vi "process speedline data.vi"(8 "Cluster in":T1={"rigChannels"=[], "rigUnits"=[], "logging"=FALSE, "chartRef"=refnum, "dataTableRef"=refnum, "channelCount"=0, "trendIndex"=0, "channels"={"massflow"=0, "PR"=0, "recircTemp"=0}, "History"={"speedlines"=[], "liveTail"={"mDot"=[], "pRatio"=[]}, "current"={"mDot"=0.0, "pRatio"=0.0}, "insertPoint"=0, "tempHistory"=[]}, "filter"=FALSE, "filterLength"=0, "tableUpdate"=0, "limitValues"=[[0.0, 45000.0], [0.0, 100.0], [0.0, 100.0], [10.0, 100.0], [0.0, 100.0], [10.0, 35.0], [0.0, 100.0], [0.0, 100.0], [99000.0, 300000.0], [-5000.0, 5000.0], [99000.0, 300000.0], [-0.01, 0.3], [-0.01, 4.5], [-0.1, 100.0], [1.0, 8.0], [1.0, 5.0], [0.0, 100.0], [0.0, 100.0], [0.0, 100.0], [-100.0, 45000.0], [-0.1, 1.0], [0.8, 2.0], [90000.0, 110000.0], [15.0, 35.0], [0.0, 0.0], [0.0, 0.0], [0.0, 0.0], [0.0, 0.0]]}, 11 "data":variant) -> (0 "Cluster out":T1={"rigChannels"=[], "rigUnits"=[], "logging"=FALSE, "chartRef"=refnum, "dataTableRef"=refnum, "channelCount"=0, "trendIndex"=0, "channels"={"massflow"=0, "PR"=0, "recircTemp"=0}, "History"={"speedlines"=[], "liveTail"={"mDot"=[], "pRatio"=[]}, "current"={"mDot"=0.0, "pRatio"=0.0}, "insertPoint"=0, "tempHistory"=[]}, "filter"=FALSE, "filterLength"=0, "tableUpdate"=0, "limitValues"=[[0.0, 45000.0], [0.0, 100.0], [0.0, 100.0], [10.0, 100.0], [0.0, 100.0], [10.0, 35.0], [0.0, 100.0], [0.0, 100.0], [99000.0, 300000.0], [-5000.0, 5000.0], [99000.0, 300000.0], [-0.01, 0.3], [-0.01, 4.5], [-0.1, 100.0], [1.0, 8.0], [1.0, 5.0], [0.0, 100.0], [0.0, 100.0], [0.0, 100.0], [-100.0, 45000.0], [-0.1, 1.0], [0.8, 2.0], [90000.0, 110000.0], [15.0, 35.0], [0.0, 0.0], [0.0, 0.0], [0.0, 0.0], [0.0, 0.0]]}, 1 "updateTable":bool, 2 "dataTable":string[][](table), 3 "plotData":cluster{"pRatio":dbl[], "mDot":dbl[]}[](array[cluster]), 4 "Recirculation Delta":dbl, 5 "temp history":dbl[][](array[numeric]))   [LabVIEW 2018]
uses:
  custom sub vis/speedlineData.ctl
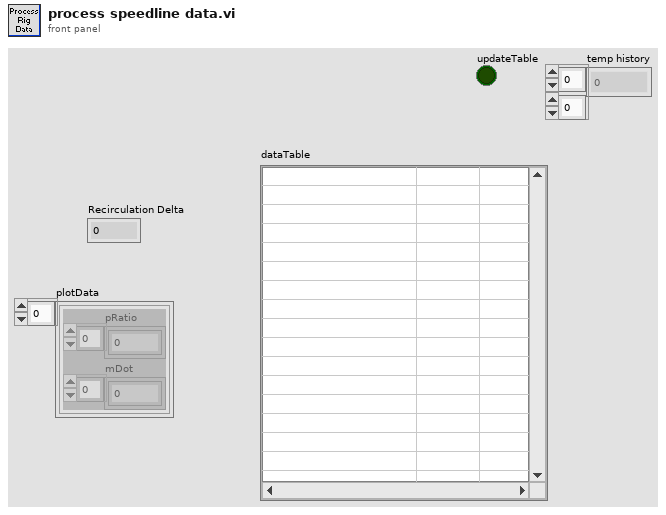
[diagram p1: front panel]
types:
  T1 = typedef "speedlineData.ctl" = cluster{"rigChannels":string[], "rigUnits":string[], "logging":bool, "chartRef":refnum<vi>, "dataTableRef":refnum<vi>, "channelCount":i32, "trendIndex":i32, "channels":cluster{"massflow":i32, "PR":i32, "recircTemp":i32}, "History":cluster{"speedlines":cluster{"mDot":dbl[], "pRatio":dbl[]}[], "liveTail":cluster{"mDot":dbl[], "pRatio":dbl[]}, "current":cluster{"mDot":dbl, "pRatio":dbl}, "insertPoint":i32, "tempHistory":dbl[][]}, "filter":bool, "filterLength":i32, "tableUpdate":i16, "limitValues":dbl[][]}
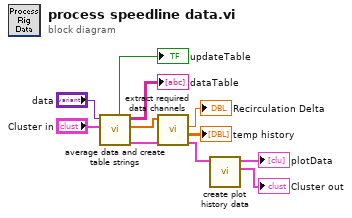
[diagram p0: block diagram]
diagram:
  n1 = call "average data and create table strings.vi"("Cluster in"="Cluster in", "rigData"="data") -> ("cluster out"=w2:T1, "averagedData"=w8:dbl[], "tableData"=→"dataTable":string[][], "updateTable"=→"updateTable":bool)  [unwired: 6 in]
  n2 = call "extract required data channels.vi"("Cluster in"=w2, "averagedData"=w8) -> ("cluster out"=w4:T1, "temp history"=→"temp history":dbl[][], "recircT"=→"Recirculation Delta":dbl)  [unwired: 7 in]
  n3 = call "create plot history data.vi"("cluster in"=w4) -> ("cluster out 2"=→"Cluster out":T1, "Array"=→"plotData":cluster{"mDot":dbl[], "pRatio":dbl[]}[])  [unwired: 9 in]
